vi "Receive message.vi"(8 "error in (no error)":errorcluster, 11 "Messenger in":refnum<class "Messenger.lvclass">) -> (0 "error out":errorcluster, 1 "new msg":bool, 2 "message":T1, 3 "Messenger out":refnum<class "Messenger.lvclass">)   [LabVIEW 2018, in "Messenger.lvclass"]
uses:
  Messenger.lvclass
  Message Queue/Message Cluster.ctl
  Messenger.lvclass/Messenger.ctl
  Message Queue/Message Queue.lvlib
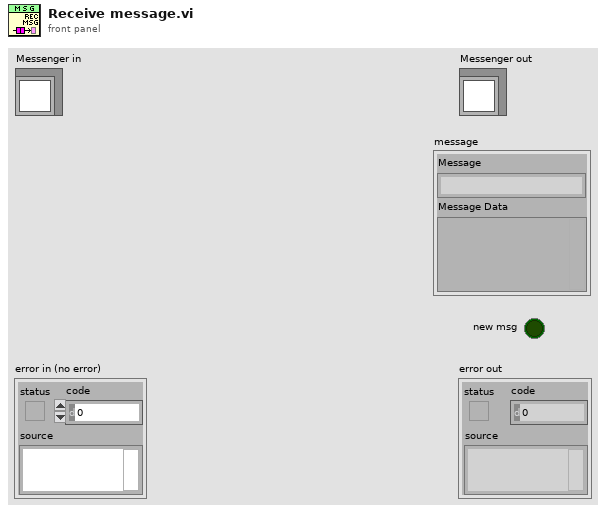
[diagram p1: front panel]
types:
  T1 = typedef "Message Queue.lvlib/Message Cluster.ctl" = cluster{"Message":string, "Message Data":variant}
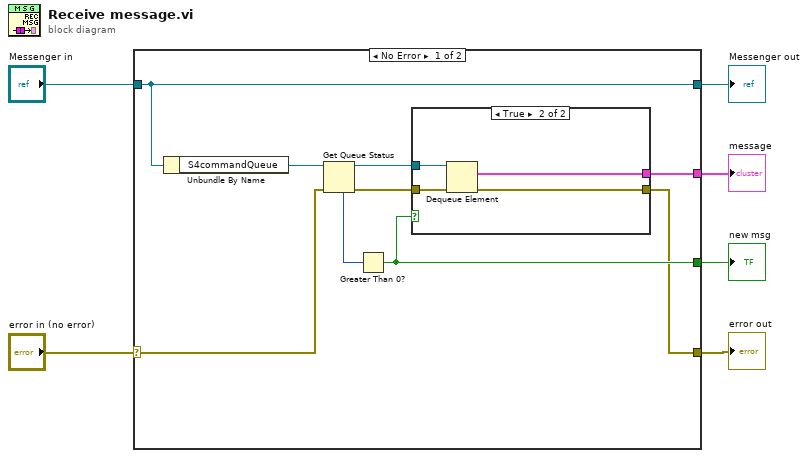
[diagram p0: block diagram]
diagram:
  n1 = case shown="No Error" "error in (no error)" {
    selector: "error in (no error)" -> [w13 w21]
    tunnel: [w8 w21] -> w5
    tunnel: [w15 w22] -> w3
    tunnel: "Messenger in" -> [w15 w22]
    tunnel: [w9 _] -> w2
    tunnel: [w7 _] -> w1
    frame No Error {
      n2 = Unbundle By Name(w15) -> ("S4commandQueue"=w14:refnum<queue>)
      n3 = Get Queue Status(queue=w14, error in (no error)=w13) -> (queue out=w10:refnum<queue>, error out=w11:errorcluster, # elements in queue=w12:i32)  [unwired: 1 in, 5 out]
      n4 = Greater Than 0?(x=w12) -> (x > 0?=w9:bool)
      n5 = case shown="True" w9 {
        tunnel: w11 -> [w16 w20]
        tunnel: w10 -> [_ w19]
        tunnel: [w16 w18] -> w8
        tunnel: [_ w17] -> w7
        frame False {
        }
        frame True {
          n6 = Dequeue Element(queue=w19, error in (no error)=w20) -> (element=w17:T1, error out=w18:errorcluster)  [unwired: 1 in, 2 out]
        }
      }
    }
    frame Error {
    }
  }
  "error out" <- w5
  "Messenger out" <- w3
  "new msg" <- w2
  "message" <- w1
